vi "Channel Load (Core).vi"(7 "Wait For Load (T)":bool=TRUE, 8 "error in (no error)":errorcluster, 9 "Path":string, 10 "Channel Index":i32, 11 "Mixer in":refnum<class "Mixer.lvclass">) -> (0 "error out":errorcluster, 3 "Mixer out":refnum<class "Mixer.lvclass">)   [LabVIEW 2020, in "G-Audio.lvlib" / "Mixer.lvclass"]
doc: "Reads an audio file into memory, and associates it with a channel.\n\nWhen <b>Wait For Load</b> is true, this VI blocks until the audio file has been loaded into a channel. If <b>Wait For Load</b> is false, this VI returns immediately and the audio file is loaded asynchronously in the background. The channel will be in a Loading state while the file is read, and then set to Loaded once the load is complete, or Empty if there was an error."
uses:
  Mixer.lvclass
  Mixer.lvclass/Mixer.ctl
  Channel/Channel.lvclass
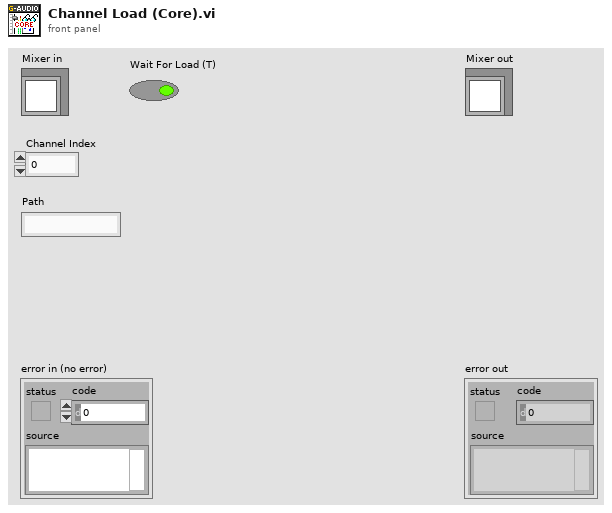
[diagram p1: front panel]
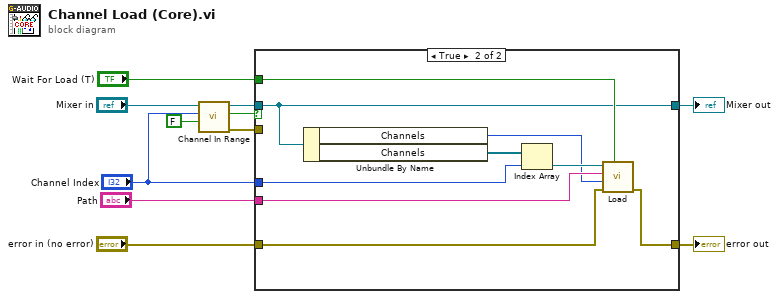
[diagram p0: block diagram]
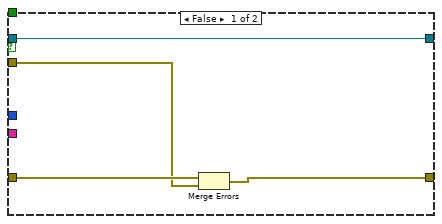
[diagram p2: hidden frame]
diagram:
  n1 = call "Channel In Range.vi"("All Channels (T)"=FALSE, "Channel Index"="Channel Index", "Mixer in"="Mixer in") -> ("error out"=w1:errorcluster, "In Range"=w2:bool, "Mixer out"=w6:refnum<class "Mixer.lvclass">)  [unwired: 6 in]
  n2 = case shown="True" w2 {
    tunnel: "Path" -> [_ w22]
    tunnel: [w12 w21] -> w10
    tunnel: "Wait For Load (T)" -> [_ w20]
    tunnel: "Channel Index" -> [_ w18]
    tunnel: w6 -> [w15 w16]
    tunnel: "error in (no error)" -> [w14 w17]
    tunnel: [w15 w16] -> w4
    tunnel: w1 -> [w13 _]
    frame False {
      n3 = Merge Errors(w14, w13) -> (w12:errorcluster)
    }
    frame True {
      n4 = Unbundle By Name(w16) -> ("Channels"=w19:u32, "Channels"=w24:refnum<data-value>[])
      n5 = Index Array(array=w24, index=w18) -> (element=w23:refnum<data-value>)
      n6 = call "Load.vi"("Wait For Load (T)"=w20, "error in (no error)"=w17, "Channels"=w19, "Path"=w22, "Channel in"=w23) -> ("error out"=w21:errorcluster)  [unwired: 5 in, 1 out]
    }
  }
  "error out" <- w10
  "Mixer out" <- w4
